vi "PolarToRect.vi"(10 "theta":dbl[](array[numeric]), 11 "r":dbl[](array[numeric])) -> (3 "Rectangular Coordinates":cluster{dbl[], dbl[]})   [LabVIEW 2020]
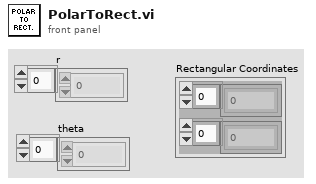
[diagram p1: front panel]
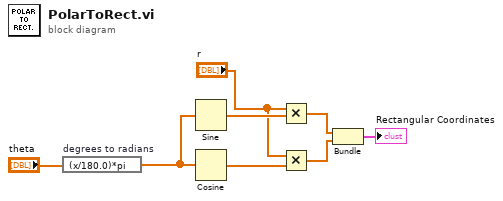
[diagram p0: block diagram]
diagram:
  n1 = expression code="(x/180.0)*pi" "degrees to radians"("theta") -> (w1:dbl[])
  n2 = Sine(x=w1) -> (sin(x)=w8:dbl[])
  n3 = Cosine(x=w1) -> (cos(x)=w6:dbl[])
  n4 = Multiply(x="r", y=w8) -> (x*y=w5:dbl[])
  n5 = Multiply(x="r", y=w6) -> (x*y=w4:dbl[])
  n6 = Bundle(w5, w4) -> (→"Rectangular Coordinates":cluster{dbl[], dbl[]})  [unwired: 1 in]
